vi "Robot Main.vi"() -> ()   [LabVIEW 2011]
doc: "This VI imlements the framework and scheduler for your robotics program. It should not be necessary to modify the framework. You are expected to add your code to the VIs called from Robot Main, the ones located in the Team Code within the project."
uses:
  <vilib>/Rock Robotics/WPI/Camera/WPI_CameraImageSize.ctl
  <vilib>/Rock Robotics/WPI/Compressor/WPI_CompressorGetSetRefNum.vi
  Robot Global Data.vi
panel:
  in  "Image Size":T1=enum."320x240"
  in  "Finish":bool
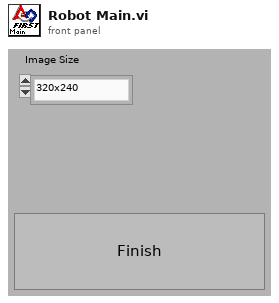
[diagram p1: front panel]
types:
  T1 = typedef "WPI_CameraImageSize.ctl" = enum16{"640x480", "320x240", "160x120"}
  T2 = typedef "WPI_CompressorDevRef.ctl" = cluster{"DevStatus":errorcluster, "DigitalInputDevRef":T3, "RelayDevRef":T6}
  T3 = typedef "WPI_DigitalInputDevRef.ctl" = cluster{"DevStatus":errorcluster, "DIO Channel":T4, "Digital Module":T5}
  T4 = typedef "FPGA_DIOChannel.ctl" = enum8{"DIO 1", "DIO 2", "DIO 3", "DIO 4", "DIO 5", "DIO 6", "DIO 7", "DIO 8", "DIO 9", "DIO 10", "DIO 11", "DIO 12", "DIO 13", "DIO 14", "Invalid"}
  T5 = typedef "FPGA_TypedefDigitalModule.ctl" = enum16{"Digital Module 1", "Digital Module 2"}
  T6 = typedef "WPI_RelayDevRef.ctl" = cluster{"DevStatus":errorcluster, "Relay Channel":T7, "Digital Module":T5, "Relay Direction":T8}
  T7 = typedef "FPGA_DIORelayChannel.ctl" = enum8{"Relay 1", "Relay 2", "Relay 3", "Relay 4", "Relay 5", "Relay 6", "Relay 7", "Relay 8", "Invalid"}
  T8 = typedef "WPI_RelayDirection.ctl" = enum16{"Both directions", "Forward only", "Reverse only"}
  T9 = typedef "WPI_DriverStationMatch Info.ctl" = cluster{"Autonomous Elapsed Seconds":dbl, "TeleOp Elapsed Seconds":dbl, "Disabled Elapsed Seconds":dbl, "Visited Autonomous":bool, "Visited TeleOp":bool, "Visited Disabled":bool, "Autonomous Settings":cluster{"Autonomous Style":enum16{"Iterative", "Independent"}, "VI Refnum":refnum<vi>}}
  T10 = typedef "WPI_DriverStationDerivedRobotMode.ctl" = enum16{"Init", "Execute", "Stop"}
  T11 = typedef "WPI_DriverStationRobotMode.ctl" = enum16{"Autonomous Disabled", "Autonomous Enabled", "Teleop Disabled", "Teleop Enabled", "Timeout", "Finish"}
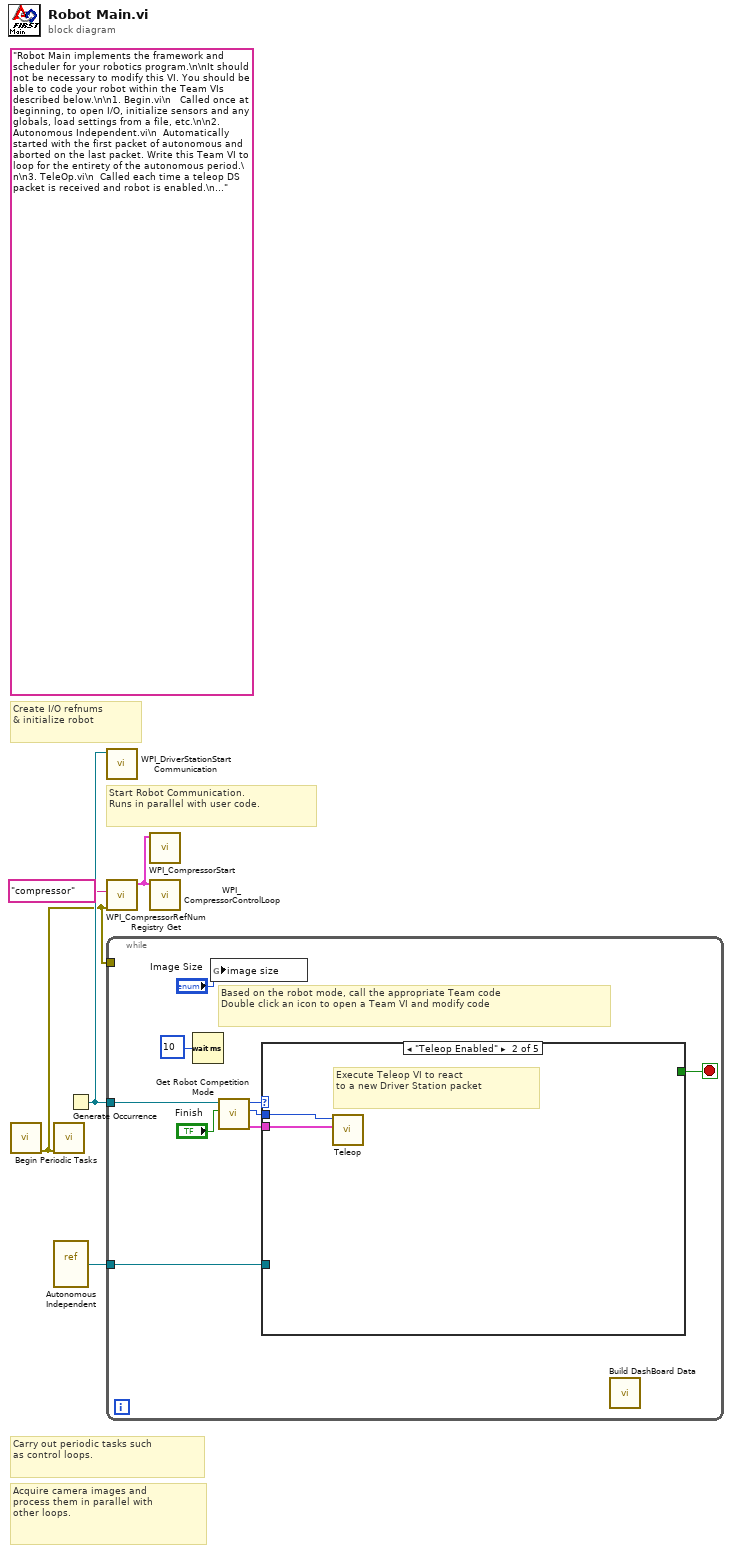
[diagram p0: block diagram]
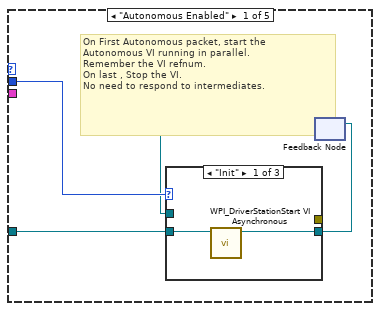
[diagram p2: hidden frame]
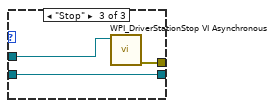
[diagram p4: hidden frame]
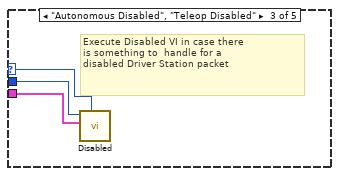
[diagram p5: hidden frame]
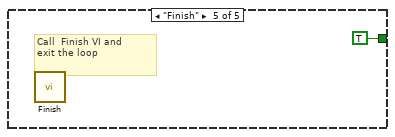
[diagram p7: hidden frame]
diagram:
  (unwired) "Robot Main implements the framework and scheduler for your robotics program.\n\nIt should not be necessary to modify this VI. You should be able to code your robot within the Team VIs described below.\n\n1. Begin.vi\n   Called once at beginning, to open I/O, initialize sensors and any globals, load settings from a file, etc.\n\n2. Autonomous Independent.vi\n  Automatically started with the first packet of autonomous and aborted on the last packet. Write this Team VI to loop for the entirety of the autonomous period.\n\n3. TeleOp.vi\n  Called each time a teleop DS packet is received and robot is enabled.\n\n4. Disabled.vi\n  Called each time a packet is received and the robot is disabled.\n\n5. Vision.vi\n  A parallel loop that acquires and processes camera images.\n\n6. PeriodicTasks.vi\n  Parallel loops running at user-defined rates.\n\n7. Finish.vi\n  Called before exiting, so you can save data, clean up I/O, etc.\n\n8. Build DashBoard Data.vi\n  Called for each driver station packet including timeouts. It is used to send select I/O values back to the Dashboard."
  # "Carry out periodic tasks such\nas control loops."
  # "Acquire camera images and\nprocess them in parallel with\nother loops."
  # "Create I/O refnums\n& initialize robot"
  # "Start Robot Communication.\nRuns in parallel with user code."
  n1 = call "Begin.vi"() -> ("error out"=w1:errorcluster)  [unwired: 1 in, 10 out]
  n2 = call "Periodic Tasks.vi"("error out"=w1) -> ()  [unwired: 1 in, 10 out]
  n3 = vi-ref "Autonomous Independent.vi"() -> (w4:refnum<vi>)
  n4 = Generate Occurrence() -> (w5:refnum<k4>)
  n5 = call <vilib>:"WPI_DriverStationStart Communication.vi"("occurrence"=w5) -> ()  [unwired: 11 out]
  n6 = call <vilib>:"WPI_CompressorRefNum Registry Get.vi"("error in (no error)"=w1, "refnum name"="compressor") -> ("CompressorDevRef"=w2:T2)  [unwired: 8 in, 1 out]
  n7 = while {
    tunnel: w5 -> [w12]
    tunnel: w4 -> [w8]
    tunnel: w1 -> [_]
    stop <- w9 stop-if-true
    # "Based on the robot mode, call the appropriate Team code\nDouble click an icon to open a Team VI and modify code"
    n8 = Wait (ms)(milliseconds to wait=u32 10) -> ()  [unwired: 1 out]
    n9 = global write "Robot Global Data.vi" "image size"("Image Size") -> ()
    n10 = call "Get Robot Competition Mode.vi"("Finish"="Finish", "DS Occurrence"=w12) -> ("Match Info out"=w10:T9, "Call Context"=w14:T10, "Robot Mode"=w13:T11)  [unwired: 7 out]
    n11 = case shown="\"Teleop Enabled\"" w13 {
      selector: w13 -> [_ _ w27 _ _]
      tunnel: w14 -> [w18 w26 w29 _ _]
      tunnel: w10 -> [_ w25 w28 _ _]
      tunnel: [_ _ _ _ TRUE] -> w9
      tunnel: w8 -> [w17 _ _ _ _]
      frame "Autonomous Enabled" {
        # "On First Autonomous packet, start the\nAutonomous VI running in parallel.\nRemember the VI refnum.\nOn last , Stop the VI.\nNo need to respond to intermediates."
        n12 = feedback #1() -> (w15:refnum<vi>)  [unwired: 1 out]
        n13 = case shown="\"Init\"" w18 {
          tunnel: w17 -> [w20 _ w23]
          tunnel: [w19 w21 w23] -> w16
          tunnel: w15 -> [_ w21 w24]
          tunnel: [_ _ w22] -> _
          frame "Init" {
            n14 = call <vilib>:"WPI_DriverStationStart VI Asynchronous.vi"("VI"=w20) -> ("VI out"=w19:refnum<vi>)  [unwired: 10 out]
          }
          frame "Execute", Default {
            # "Nothing to do"
          }
          frame "Stop" {
            n15 = call <vilib>:"WPI_DriverStationStop VI Asynchronous.vi"("VI Refnum"=w24) -> ("error out"=w22:errorcluster)  [unwired: 10 out]
          }
        }
        n16 = feedback-in #1(w16) -> ()
      }
      frame "Teleop Enabled" {
        # "Execute Teleop VI to react\nto a new Driver Station packet"
        n17 = call "Teleop.vi"("Match Info"=w25, "Call Context"=w26) -> ()  [unwired: 1 in, 9 out]
      }
      frame "Autonomous Disabled", "Teleop Disabled" {
        # "Execute Disabled VI in case there\nis something to  handle for a\ndisabled Driver Station packet"
        n18 = call "Disabled.vi"("Robot Mode"=w27, "Match Info"=w28, "Call Context"=w29) -> ()  [unwired: 1 in, 8 out]
      }
      frame "Timeout" {
        # "Driver Station packet didn't arrive.\nPossibly useful for diagnostics"
      }
      frame "Finish" {
        # "Call  Finish VI and\nexit the loop"
        n19 = call "Finish.vi"() -> ()  [unwired: 1 in, 7 out]
      }
    }
    n20 = call "Build DashBoard Data.vi"() -> ()  [unwired: 1 in, 11 out]
  }
  n21 = call <vilib>:"WPI_CompressorStart.vi"("CompressorDevRef"=w2) -> ()  [unwired: 9 in, 2 out]
  n22 = call <vilib>:"WPI_CompressorControlLoop.vi"("CompressorDevRef"=w2) -> ()  [unwired: 11 in]
